vi "Teleop.vi"(9 "output cluster":T1, 10 "Match Info":T2={"Autonomous Elapsed Seconds"=0.0, "TeleOp Elapsed Seconds"=0.0, "Disabled Elapsed Seconds"=0.0, "Visited Autonomous"=FALSE, "Visited TeleOp"=FALSE, "Visited Disabled"=FALSE, "Autonomous Settings"={"Autonomous Style"=enum."Independent", "VI Refnum"=refnum}}, 11 "Call Context":T3) -> (1 "output cluster 2":T1)   [LabVIEW 2017]
doc: "This VI is called for each TeleOp packet received from the DS where the robot is not disabled. It is often used to read from the joysticks and update I/O or to update setpoints for timed control loops. It should complete and return within 20 milliseconds or it may miss DS packets."
uses:
  <vilib>/Rock Robotics/WPI/DriverStation/WPI_DriverStationDerivedRobotMode.ctl
  <vilib>/Rock Robotics/WPI/DriverStation/WPI_DriverStationMatch Info.ctl
  Drive/Classes.ctl
  Drive/Drive.lvclass
  <vilib>/Rock Robotics/Network Tables/NT Read Number.vi
  <vilib>/Rock Robotics/WPI/Utilities/WPI_GetSetVariantRefNum.vi
  <vilib>/Rock Robotics/Network Tables/NT Write Boolean Array.vi
  <vilib>/Rock Robotics/Network Tables/NT Write Numeric Array.vi
  <vilib>/Rock Robotics/Network Tables/NT Read Boolean.vi
  <vilib>/gmath/NI_Gmath.lvlib
panel:
  out "x-y":dbl
  out "Waveform Chart":u32(graph)
  in  "error in (no error)":errorcluster
  out "Sample Slider 0":dbl(slide) scale=0.0..5.0
  out "Sample Boolean 1":bool
  out "Sample Boolean 0":bool
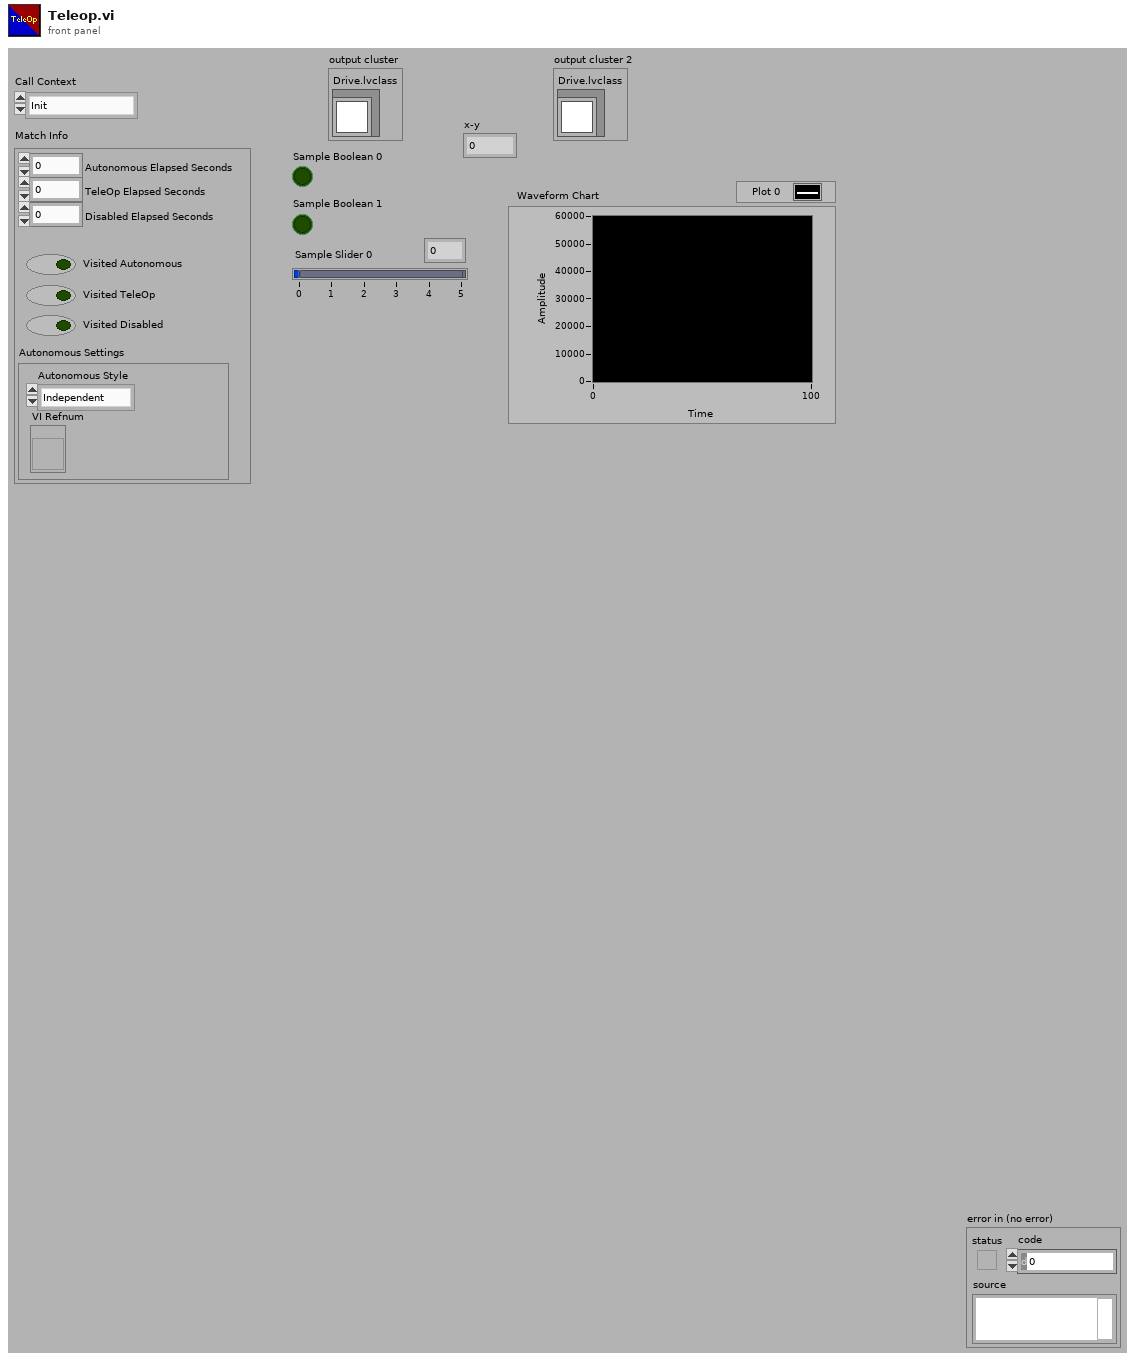
[diagram p1: front panel]
types:
  T1 = typedef "Classes.ctl" = cluster{"Drive.lvclass":refnum<class "Drive.lvclass">}
  T2 = typedef "WPI_DriverStationMatch Info.ctl" = cluster{"Autonomous Elapsed Seconds":dbl, "TeleOp Elapsed Seconds":dbl, "Disabled Elapsed Seconds":dbl, "Visited Autonomous":bool, "Visited TeleOp":bool, "Visited Disabled":bool, "Autonomous Settings":cluster{"Autonomous Style":enum16{"Iterative", "Independent"}, "VI Refnum":refnum<vi>}}
  T3 = typedef "WPI_DriverStationDerivedRobotMode.ctl" = enum16{"Init", "Execute", "Stop"}
  T4 = cluster{"offsetAngle H":dbl, "offsetAngle V":dbl, "area":dbl, "skew":dbl, "target":dbl}
  T5 = typedef "WPI_MotorControlDeviceRef.ctl" = cluster{"DeviceStatus":errorcluster, "Type":T6, "PWM":cluster{"PWM Channel":T7, "DeadBand":T8}, "CAN":cluster{"Device Number":u8, "SetOutput VI Ref":variant, "GetOutput VI Ref":variant, "Enable VI Ref":variant, "Disable VI Ref":variant, "Data":variant}, "Invert":bool, "DIO PWM":cluster{"PWM \"Enable\" Channel":T7, "DIOChannel":T9, "PWM Rate":dbl}}
  T6 = typedef "WPI_MotorControlType.ctl" = enum16{"PWM", "CAN", "DIO PWM"}
  T7 = typedef "FPGA_DIOPWMChannel.ctl" = enum8{"PWM 0", "PWM 1", "PWM 2", "PWM 3", "PWM 4", "PWM 5", "PWM 6", "PWM 7", "PWM 8", "PWM 9", "PWM MXP 0", "PWM MXP 1", "PWM MXP 2", "PWM MXP 3", "PWM MXP 4", "PWM MXP 5", "PWM MXP 6", "PWM MXP 7", "PWM MXP 8", "PWM MXP 9", "Invalid"}
  T8 = typedef "WPI_PWMDeadband.ctl" = cluster{"Name":string, "maxPositivePwm":i32, "minPositivePwm":i32, "centerPwm":i32, "maxNegativePwm":i32, "minNegativePwm":i32, "angularRange":u16}
  T9 = typedef "FPGA_DIOChannel.ctl" = enum8{"DIO 0", "DIO 1", "DIO 2", "DIO 3", "DIO 4", "DIO 5", "DIO 6", "DIO 7", "DIO 8", "DIO 9", "DIO MXP 0", "DIO MXP 1", "DIO MXP 2", "DIO MXP 3", "DIO MXP 4", "DIO MXP 5", "DIO MXP 6", "DIO MXP 7", "DIO MXP 8", "DIO MXP 9", "DIO MXP 10", "DIO MXP 11", "DIO MXP 12", "DIO MXP 13", "DIO MXP 14", "DIO MXP 15", "SPI Port CS1", "SPI Port CS2", "SPI Port CS3", "SPI Port MISO", "SPI Port MOSI", "Invalid"}
  T10 = typedef "WPI_JoystickDevRef.ctl" = cluster{"Device":T11}
  T11 = typedef "WPI_JoystickDeviceEnum.ctl" = enum16{"USB 0", "USB 1", "USB 2", "USB 3", "USB 4", "USB 5"}
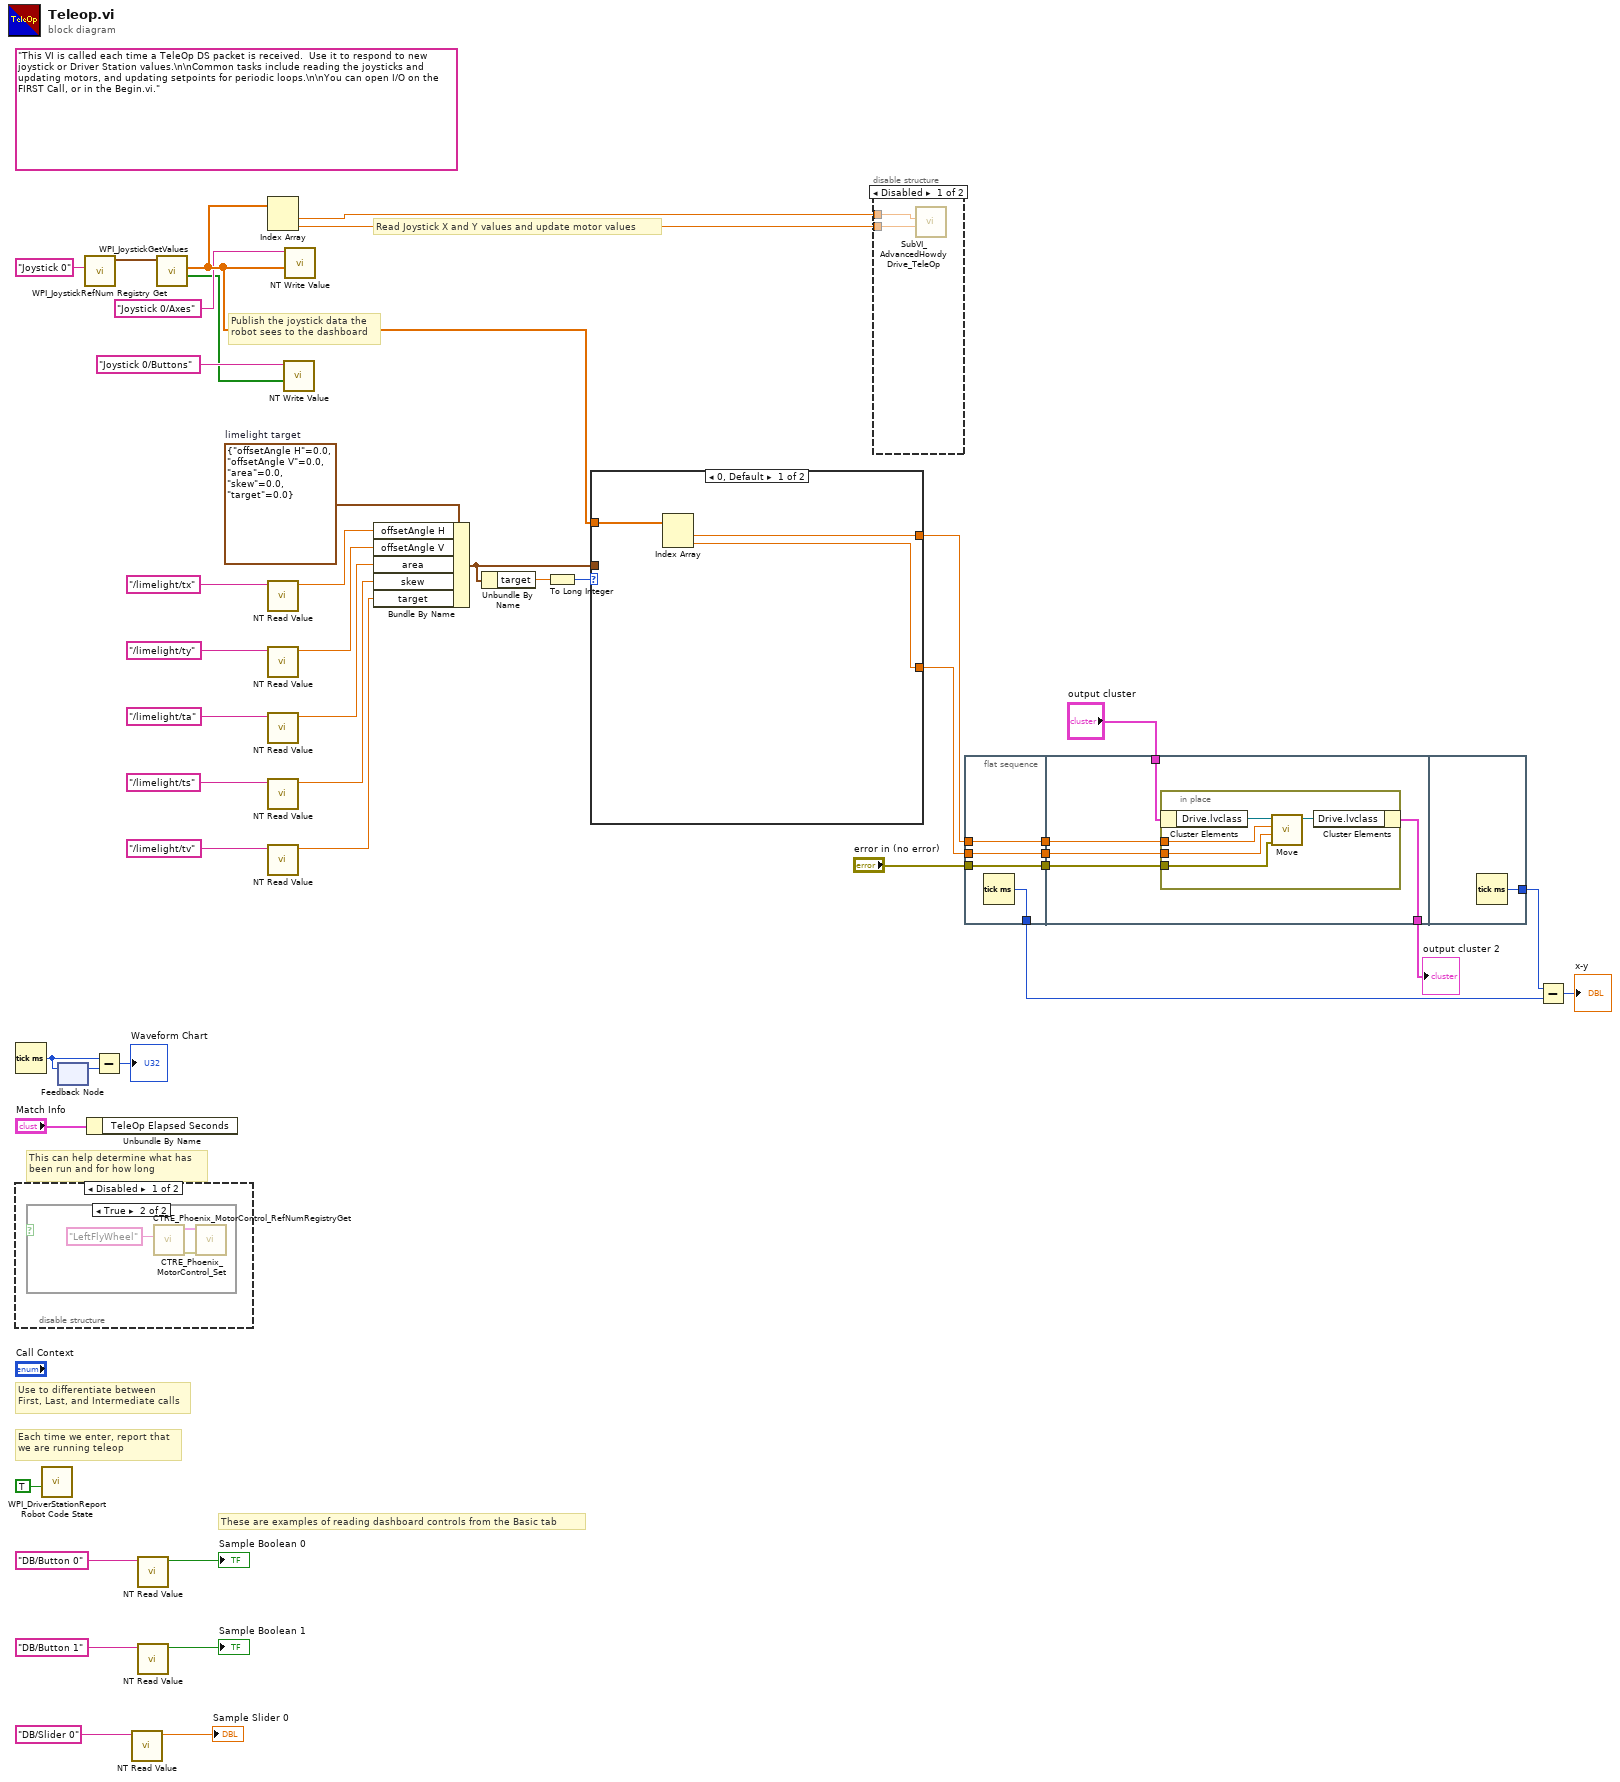
[diagram p0: block diagram]
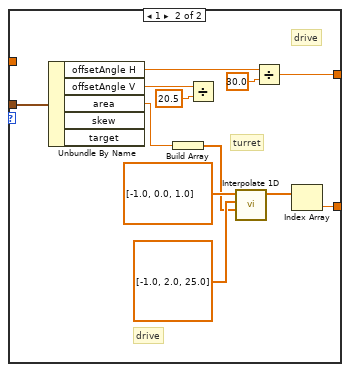
[diagram p4: hidden frame]
diagram:
  w32 = T4 {"offsetAngle H"=0.0, "offsetAngle V"=0.0, "area"=0.0, "skew"=0.0, "target"=0.0}  # limelight target
  (unwired) "This VI is called each time a TeleOp DS packet is received.  Use it to respond to new joystick or Driver Station values.\n\nCommon tasks include reading the joysticks and updating motors, and updating setpoints for periodic loops.\n\nYou can open I/O on the FIRST Call, or in the Begin.vi."
  # "These are examples of reading dashboard controls from the Basic tab"
  # "Each time we enter, report that\nwe are running teleop"
  # "Use to differentiate between\nFirst, Last, and Intermediate calls"
  # "This can help determine what has\nbeen run and for how long"
  # "Read Joystick X and Y values and update motor values"
  # "Publish the joystick data the\nrobot sees to the dashboard"
  n1 = Tick Count (ms)() -> (millisecond timer value=w5:u32)
  n2 = disable-structure shown="Disabled" {
    frame Disabled {
      n3 = case shown="True" {
        selector: _ -> [_ _]
        frame False {
        }
        frame True {
          n4 = call <vilib>:"CTRE_Phoenix_MotorControl_RefNumRegistryGet.vi"("refnum name"="LeftFlyWheel") -> ("error out"=w46:errorcluster, "PhoenixMotorControlDevRef"=w45:T5)  [unwired: 9 in]
          n5 = call <vilib>:"CTRE_Phoenix_MotorControl_Set.vi"("error in (no error)"=w46, "PhoenixMotorControlDevRef"=w45) -> ()  [unwired: 8 in, 2 out]
        }
      }
    }
    frame Enabled {
    }
  }
  n6 = call <vilib>:"WPI_DriverStationReport Robot Code State.vi"("TeleOp"=TRUE ("Autonomous")) -> ()  [unwired: 10 in, 1 out]
  n7 = feedback #1() -> (w4:u32)  [unwired: 1 in]
  n8 = feedback-in #1(w5) -> ()
  n9 = call <vilib>:"WPI_JoystickRefNum Registry Get.vi"("refnum name"="Joystick 0") -> ("JoystickDevRef"=w17:T10)  [unwired: 1 in, 9 out]
  n10 = Unbundle By Name("Match Info") -> ()  [unwired: 1 out]
  n11 = Subtract(x=w5, y=w4) -> (x-y=→"Waveform Chart":u32)
  n12 = call-poly <vilib>:"NT Read Value.vi"("Name"="DB/Slider 0" ("refnum name")) -> ("Numeric"=→"Sample Slider 0":dbl)  [unwired: 9 in, 1 out]
  n13 = call-poly <vilib>:"NT Read Value.vi"("Name"="DB/Button 0" ("refnum name")) -> ("Boolean"=→"Sample Boolean 0":bool)  [unwired: 9 in, 1 out]
  n14 = call-poly <vilib>:"NT Read Value.vi"("Name"="DB/Button 1" ("refnum name")) -> ("Boolean"=→"Sample Boolean 1":bool)  [unwired: 9 in, 1 out]
  n15 = call <vilib>:"WPI_JoystickGetValues.vi"("JoystickDevRef"=w17) -> ("Buttons"=w14:bool[], "Axes"=w39:dbl[])  [unwired: 6 in, 3 out]
  n16 = Index Array(array=w39) -> (element #1=w44:dbl, element #2=w43:dbl)  [unwired: 2 in]
  n17 = call-poly <vilib>:"NT Read Value.vi"("Name"="/limelight/tx") -> ("Numeric"=w31:dbl)  [unwired: 9 in, 1 out]
  n18 = call-poly <vilib>:"NT Read Value.vi"("Name"="/limelight/ty") -> ("Numeric"=w25:dbl)  [unwired: 9 in, 1 out]
  n19 = call-poly <vilib>:"NT Read Value.vi"("Name"="/limelight/ta") -> ("Numeric"=w30:dbl)  [unwired: 9 in, 1 out]
  n20 = call-poly <vilib>:"NT Read Value.vi"("Name"="/limelight/ts") -> ("Numeric"=w29:dbl)  [unwired: 9 in, 1 out]
  n21 = call-poly <vilib>:"NT Read Value.vi"("Name"="/limelight/tv") -> ("Numeric"=w28:dbl)  [unwired: 9 in, 1 out]
  n22 = call-poly <vilib>:"NT Write Value.vi"("Boolean Array"=w14, "Name"="Joystick 0/Buttons") -> ()  [unwired: 9 in, 1 out]
  n23 = call-poly <vilib>:"NT Write Value.vi"("Numeric Array"=w39, "Name"="Joystick 0/Axes") -> ()  [unwired: 9 in, 1 out]
  n24 = Bundle By Name(cluster=w32, "offsetAngle H"=w31, "offsetAngle V"=w25, "area"=w30, "skew"=w29, "target"=w28) -> (w26:T4)
  n25 = Unbundle By Name(w26) -> ("target"=w27:dbl)
  n26 = To Long Integer(number=w27) -> (32bit integer=w19:i32)
  n27 = case shown="0, Default" w19 {
    tunnel: w26 -> [_ w62]
    tunnel: [w49 w51] -> w41
    tunnel: [w50 w52] -> w42
    tunnel: w39 -> [w48 _]
    frame 0, Default {
      n28 = Index Array(array=w48) -> (element #1=w50:dbl, element #2=w49:dbl)  [unwired: 2 in]
    }
    frame 1 {
      # "drive"
      # "drive"
      # "turret"
      n29 = Unbundle By Name(w62) -> ("offsetAngle H"=w61:dbl, "offsetAngle V"=w59:dbl, "area"=w55:dbl)  [unwired: 2 out]
      n30 = Build Array(w55) -> (w54:dbl[])
      n31 = Divide(x=w59, y=20.5) -> ()  [unwired: 1 out]
      n32 = call <vilib>:"Interpolate 1D.vi"("xi"=w54, "X"=dbl[] [-1.0, 2.0, 25.0], "Y"=dbl[] [-1.0, 0.0, 1.0]) -> ("yi"=w53:dbl[])  [unwired: 6 in, 2 out]
      n33 = Divide(x=w61, y=30.0) -> (x/y=w52:dbl)
      n34 = Index Array(array=w53) -> (element=w51:dbl)  [unwired: 1 in]
    }
  }
  n35 = disable-structure shown="Disabled" {
    disable-tunnel: w44 -> [w64 _]
    disable-tunnel: w43 -> [w63 _]
    frame Disabled {
      n36 = call "SubVI_AdvancedHowdyDrive_TeleOp.vi"("Y axis value"=w63, "X axis value"=w64) -> ()  [unwired: 8 in, 2 out]
    }
    frame Enabled {
    }
  }
  n37 = flat-sequence {
    tunnel: "error in (no error)" -> [w66]
    tunnel: w41 -> [w67]
    tunnel: w42 -> [w68]
    tunnel: [w68] -> w38
    tunnel: [w67] -> w37
    tunnel: [w66] -> w36
    tunnel: [w65] -> w34
    tunnel: w38 -> [w73]
    tunnel: w37 -> [w72]
    tunnel: w36 -> [w71]
    tunnel: "output cluster" -> [w70]
    tunnel: [w69] -> w1
    tunnel: [w79] -> w33
    frame #0 {
      n38 = Tick Count (ms)() -> (millisecond timer value=w65:u32)
    }
    frame #1 {
      n39 = in-place {
        in-place-border: w73 -> [w78]
        in-place-border: w72 -> [w77]
        in-place-border: w71 -> [w76]
        n40 = in-place-cluster #2(w70) -> ("Drive.lvclass"=w75:refnum<class "Drive.lvclass">)
        n41 = call-dynamic "Move.vi"("error in (no error)"=w76, "Y"=w77, "X"=w78, "Drive in"=w75) -> ("Drive out"=w74:refnum<class "Drive.lvclass">)  [unwired: 6 in, 1 out]
        n42 = in-place-cluster #2("Drive.lvclass"=w74) -> (w69:T1)
      }
    }
    frame #2 {
      n43 = Tick Count (ms)() -> (millisecond timer value=w79:u32)
    }
  }
  n44 = Subtract(x=w33, y=w34) -> (x-y=→"x-y":u32)
  "output cluster 2" <- w1
